vi "A x B.vi"   [LabVIEW 2017, in "NI_AALBase.lvlib"]
doc: "Performs the multiplication of two input matrices or an input matrix and an input vector. The data types you wire to the <B>A</B> and <B>B</B> inputs determine the polymorphic instance to use."
uses:
  <vilib>/Analysis/NI_AALBase.lvlib
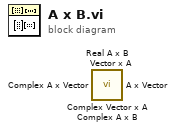
[diagram p0: block diagram]
diagram:
  n1 = call <vilib>:"Complex Vector x A.vi"() -> ()  [unwired: 2 in, 2 out]
  n2 = call <vilib>:"Vector x A.vi"() -> ()  [unwired: 2 in, 2 out]
  n3 = call <vilib>:"Complex A x Vector.vi"() -> ()  [unwired: 2 in, 2 out]
  n4 = call <vilib>:"A x Vector.vi"() -> ()  [unwired: 2 in, 2 out]
  n5 = call <vilib>:"Complex A x B.vi"() -> ()  [unwired: 2 in, 2 out]
  n6 = call <vilib>:"Real A x B.vi"() -> ()  [unwired: 2 in, 2 out]
